vi "HW_GEN - Config Tree Dis Colums.vi"(11 "ActiveModu.CHtype":string) -> (3 "ColInfo":T1)   [LabVIEW 2016]
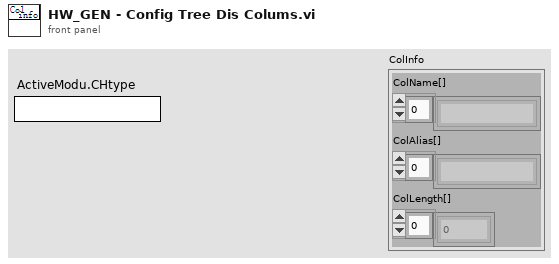
[diagram p1: front panel]
types:
  T1 = cluster{"ColName[]":string[], "ColAlias[]":string[], "ColLength[]":i32[]}
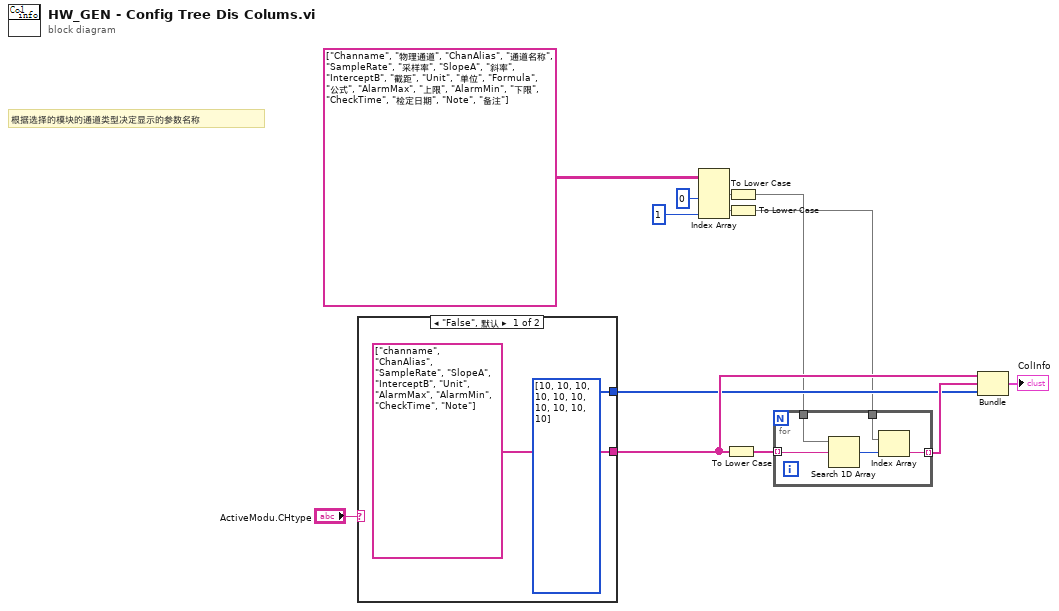
[diagram p0: block diagram]
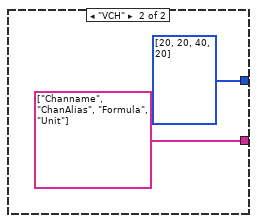
[diagram p2: hidden frame]
diagram:
  # "根据选择的模块的通道类型决定显示的参数名称"
  n1 = case shown="\"False\", 默认" "ActiveModu.CHtype" {
    tunnel: [string[] ["channame", "ChanAlias", "SampleRate", "SlopeA", "InterceptB", "Unit", "AlarmMax", "AlarmMin", "CheckTime", "Note"] ("transposed array") string[] ["Channame", "ChanAlias", "Formula", "Unit"] ("DisCols[]")] -> w7
    tunnel: [i32[] [10, 10, 10, 10, 10, 10, 10, 10, 10, 10] i32[] [20, 20, 40, 20]] -> w5
    frame "False", Default {
    }
    frame "VCH" {
    }
  }
  n2 = Index Array(array=string[][] [["Channame", "物理通道"], ["ChanAlias", "通道名称"], ["SampleRate", "采样率"], ["SlopeA", "斜率"], ["InterceptB", "截距"], ["Unit", "单位"], ["Formula", "公式"], ["AlarmMax", "上限"], ["AlarmMin", "下限"], ["CheckTime", "检定日期"], ["Note", "备注"]] ("DisCols[]"), index (col) #1=0 ("disabled index (col)"), index (col) #2=1 ("index (col)")) -> (element #1=w9:string[], element #2=w8:string[])  [unwired: 2 in]
  n3 = To Lower Case(string=w7) -> (all lower case string=w1:string[])
  n4 = To Lower Case(string=w9) -> (all lower case string=w3:string[])
  n5 = To Lower Case(string=w8) -> (all lower case string=w2:string[])
  n6 = for {
    tunnel: w1 -> [w21] mode=indexing
    tunnel: w3 -> [w22]
    tunnel: w2 -> [w19]
    tunnel: [w18] -> w6 mode=indexing
    n7 = Search 1D Array(1D array=w22, element=w21) -> (index of element=w20:i32)  [unwired: 1 in]
    n8 = Index Array(array=w19, index=w20) -> (element=w18:string)
  }
  n9 = Bundle("DisCols[]"=w7, w6, w5) -> (→"ColInfo":cluster{"DisCols[]":string[], string[], i32[]})  [unwired: 1 in]
